vi "Main.vi"() -> ()   [LabVIEW 2020]
doc: "Use this template to build a simple state machine design pattern. Each state executes code and determines which state to transition to."
uses:
  controls/StateMachineVariables.ctl
  <vilib>/vision/Avi.llb/IMAQ AVI2 Refnum.ctl
  <vilib>/userDefined/High Color/IMAQdx.ctl
  <vilib>/vision/Deep Learning.llb/IMAQ DL Model Refnum.ctl
  <vilib>/vision/Image Controls.llb/IMAQ Image.ctl
  controls/State.ctl
panel:
  in  "Cluster":T1
  in  "Turn on the replay mode":bool=TRUE
  out "Replay mode":bool
  in  "?":T6(tab)
  in  "Camera Name":refnum<k21> caption="IMAQdx Session"
  out "fps cam":dbl
  out "height":u32
  out "width":u32
  in  "Start Frame Number":u32
  out "Actual frame":u32
  in  "Frame increment":i32=1
  in  "Video fps":u32=30
  in  "Video filename":string="test_moving2.avi"
  in  "Height":i32=1080
  in  "Width":i32=1920
  out "fps detection":dbl
  out "Distance":sgl(graph)
  # "SWITCH MODE BETWEEN\nCAMERA OR REPLAY"
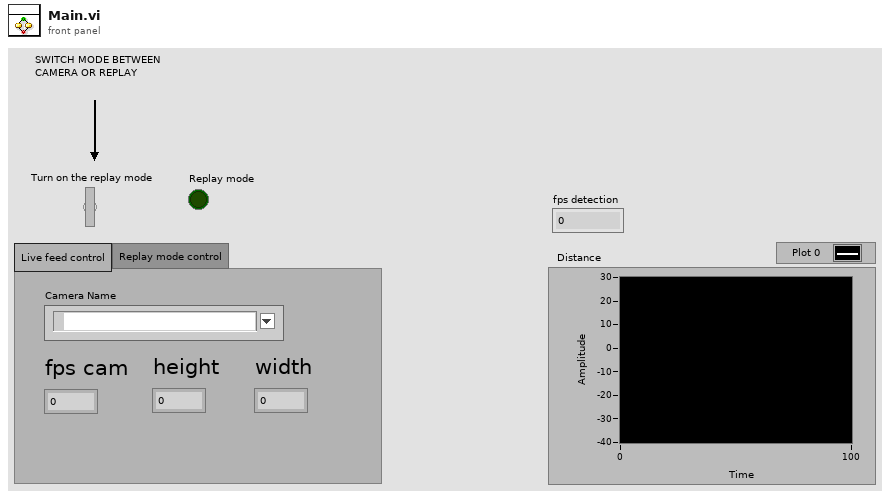
[diagram p1: front panel]
types:
  T1 = typedef "StateMachineVariables.ctl" = cluster{"AVI Refnum":T2, "Session ID":T3, "TensorFlow model refnum":T4, "Image refnum":T5, "VI path":path, "Horizontal distance":dbl, "Lateral distance":dbl, "Relative speed":dbl, "FPS":dbl}
  T2 = typedef "IMAQ AVI2 Refnum.ctl" = refnum<k20>
  T3 = typedef "IMAQdx.ctl" = refnum<k21>
  T4 = typedef "IMAQ DL Model Refnum.ctl" = refnum<k20>
  T5 = typedef "IMAQ Image.ctl" = refnum<image>
  T6 = enum32{"Live feed control", "Replay mode control"}
  T7 = typedef "State.ctl" = enum16{"Initialize VI path", "Initialize Video Session", "Initialize Cam session", "Initialize TensorFlow Model", "Initialize Image refnum", "Get video frame", "Get Cam frame", "Analyze image", "Update reaction space"}
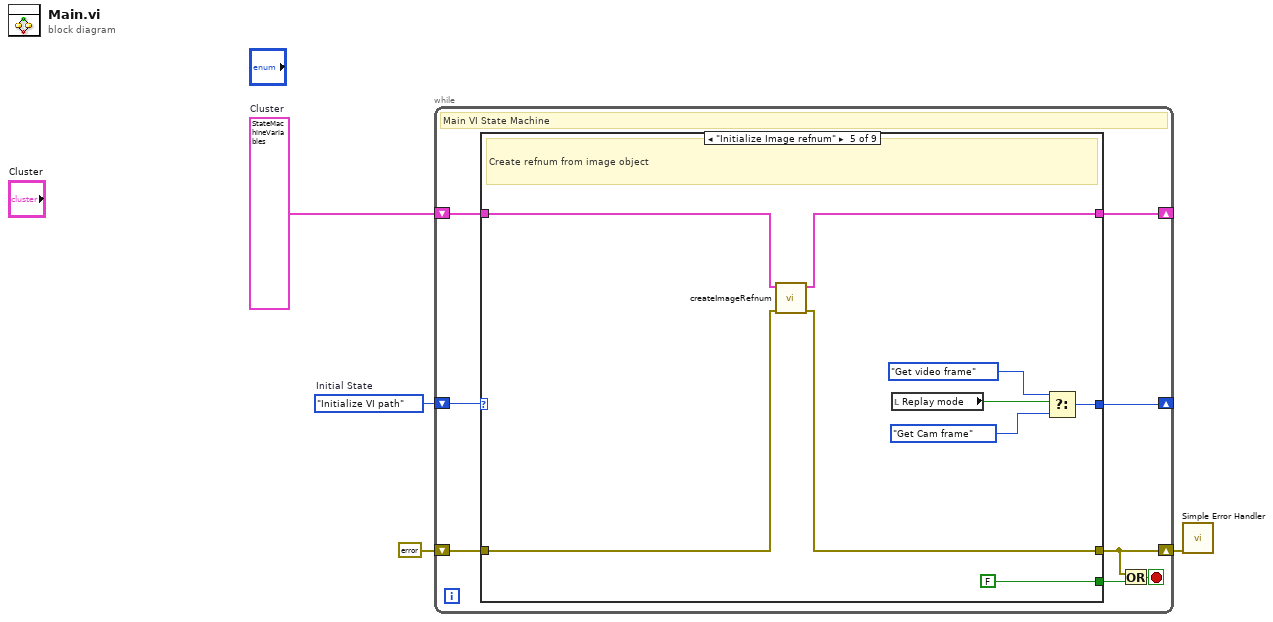
[diagram p0: block diagram]
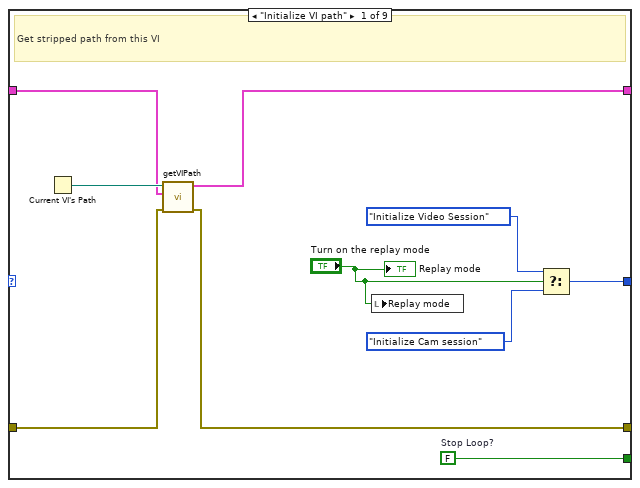
[diagram p2: hidden frame]
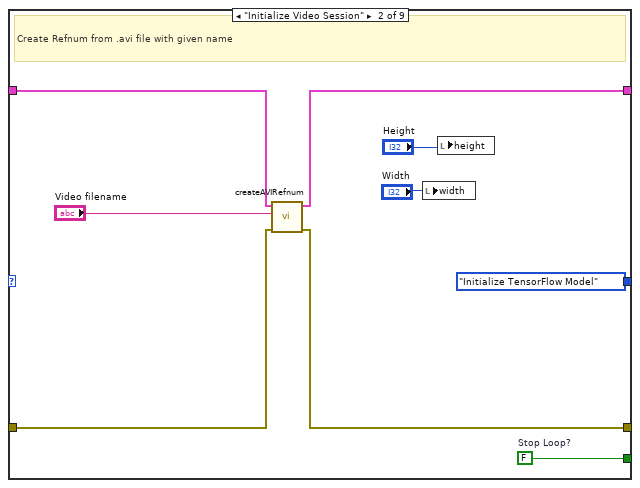
[diagram p3: hidden frame]
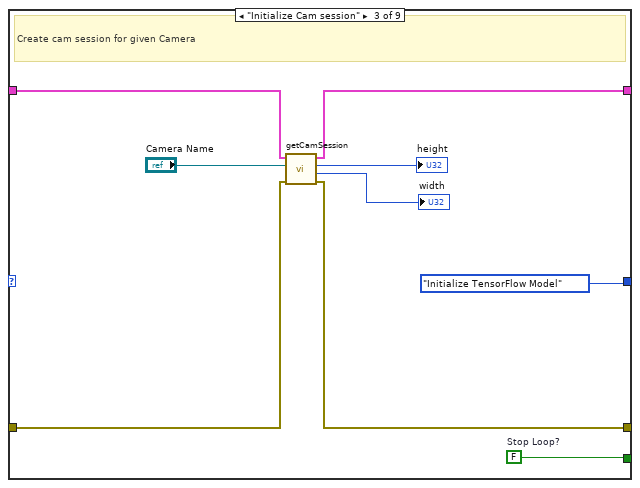
[diagram p4: hidden frame]
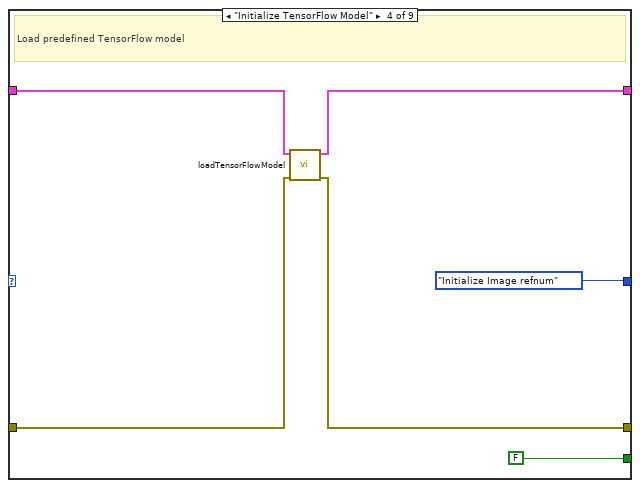
[diagram p5: hidden frame]
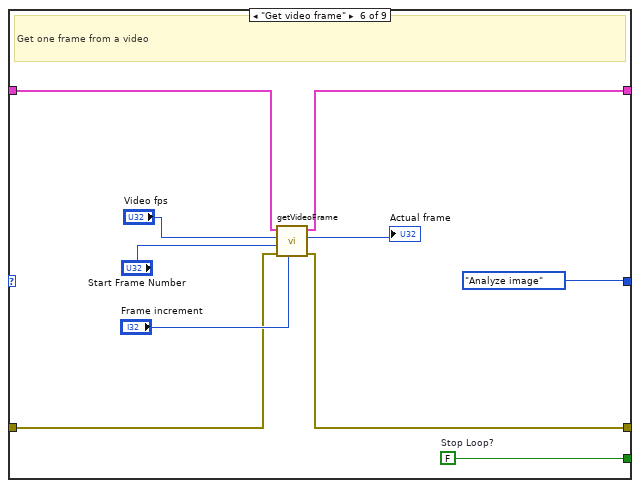
[diagram p6: hidden frame]
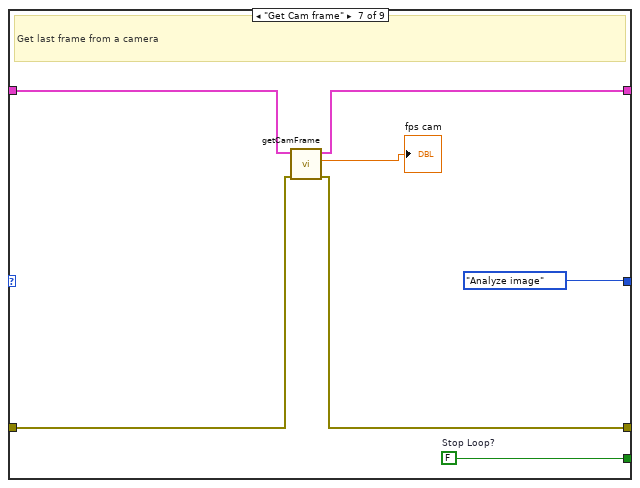
[diagram p7: hidden frame]
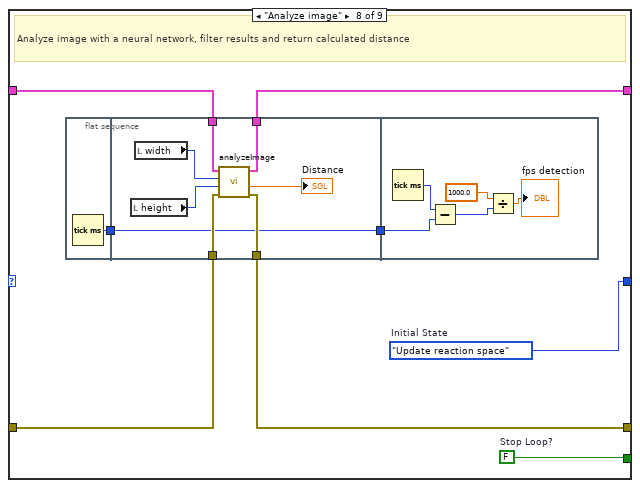
[diagram p8: hidden frame]
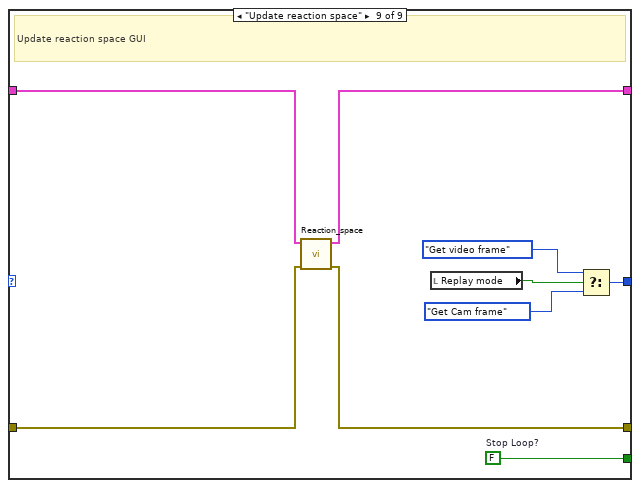
[diagram p9: hidden frame]
diagram:
  w2 = T1 {"AVI Refnum"=refnum, "Session ID"="", "TensorFlow model refnum"=refnum, "Image refnum"=refnum, "VI path"=path "", "Horizontal distance"=0.0, "Lateral distance"=0.0, "Relative speed"=0.0, "FPS"=0.0}  # Cluster
  w1 = State."Initialize VI path"  # Initial State
  n1 = while {
    shift-right: [w11] -> _
    shift-left: w2 -> [w12]
    shift-right: [w5] -> w3
    shift-left: errorcluster {"status"=FALSE, "code"=0, "source"=""} ("error constant") -> [w10]
    shift-right: [w7] -> _
    shift-left: w1 -> [w6]
    stop <- w8 stop-if-true
    # "Main VI State Machine"
    n2 = case shown="\"Initialize Image refnum\"" w6 {
      tunnel: [w15 State."Initialize TensorFlow Model" State."Initialize TensorFlow Model" State."Initialize Image refnum" w47 State."Analyze image" State."Analyze image" w75 w96] -> w7
      tunnel: [w22 w31 w34 FALSE ("Stop Loop?") FALSE ("Stop Loop?") w65 w67 w76 w99] -> w9
      tunnel: w12 -> [w20 w26 w39 w44 w54 w58 w72 w80 w103]
      tunnel: [w19 w25 w38 w43 w53 w59 w66 w79 w102] -> w11
      tunnel: w10 -> [w17 w24 w37 w41 w51 w60 w70 w78 w101]
      tunnel: [w18 w23 w36 w42 w52 w61 w69 w77 w100] -> w5
      frame "Initialize VI path" {
        w22 = FALSE  # Stop Loop?
        # "Get stripped path from this VI"
        n3 = Current VI's Path() -> (path=w21:path)
        n4 = call "getVIPath.vi"("error in"=w17, "Cluster in"=w20, "path"=w21) -> ("error out"=w18:errorcluster, "Cluster out"=w19:T1)  [unwired: 7 in]
        n5 = local write "Replay mode"("Turn on the replay mode") -> ()
        n6 = Select(t=State."Initialize Video Session", s="Turn on the replay mode", f=State."Initialize Cam session") -> (s? t:f=w15:T7)
        "Replay mode" <- "Turn on the replay mode"
      }
      frame "Initialize Video Session" {
        w31 = FALSE  # Stop Loop?
        # "Create Refnum from .avi file with given name"
        n7 = call "createAVIRefnum.vi"("error in"=w24, "Video filename"="Video filename", "Input cluster"=w26) -> ("error out"=w23:errorcluster, "Output cluster"=w25:T1)  [unwired: 7 in]
        n8 = local write "width"("Width") -> ()
        n9 = local write "height"("Height") -> ()
      }
      frame "Initialize Cam session" {
        w34 = FALSE  # Stop Loop?
        # "Create cam session for given Camera"
        n10 = call "getCamSession.vi"("error in"=w37, "Camera name"="Camera Name", "Input cluster"=w39) -> ("error out"=w36:errorcluster, "Width"=→"width":u32, "Height"=→"height":u32, "Output cluster"=w38:T1)  [unwired: 5 in]
      }
      frame "Initialize TensorFlow Model" {
        # "Load predefined TensorFlow model"
        n11 = call "loadTensorFlowModel.vi"("error in"=w41, "Input cluster"=w44) -> ("error out"=w42:errorcluster, "Output cluster"=w43:T1)  [unwired: 8 in]
      }
      frame "Initialize Image refnum" {
        # "Create refnum from image object"
        n12 = call "createImageRefnum.vi"("error in"=w51, "Output cluster in"=w54) -> ("error out"=w52:errorcluster, "Output cluster out"=w53:T1)  [unwired: 8 in]
        n13 = local read "Replay mode"() -> (w48:bool)
        n14 = Select(t=State."Get video frame", s=w48, f=State."Get Cam frame") -> (s? t:f=w47:T7)
      }
      frame "Get video frame" {
        w65 = FALSE  # Stop Loop?
        # "Get one frame from a video"
        n15 = call "getVideoFrame.vi"("Frame increment"="Frame increment", "error in (no error)"=w60, "Start Frame Number"="Start Frame Number", "Video fps"="Video fps", "Input cluster"=w58) -> ("error out"=w61:errorcluster, "Actual frame"=→"Actual frame":u32, "Output cluster"=w59:T1)  [unwired: 4 in]
      }
      frame "Get Cam frame" {
        w67 = FALSE  # Stop Loop?
        # "Get last frame from a camera"
        n16 = call "getCamFrame.vi"("error in (no error)"=w70, "Cluster"=w72) -> ("error out"=w69:errorcluster, "Acquired Frames per Second"=→"fps cam":dbl, "output cluster"=w66:T1)  [unwired: 7 in]
      }
      frame "Analyze image" {
        w76 = FALSE  # Stop Loop?
        w75 = State."Update reaction space"  # Initial State
        # "Analyze image with a neural network, filter results and return calculated distance"
        n17 = flat-sequence {
          tunnel: [w81] -> w74
          tunnel: w80 -> [w89]
          tunnel: [w88] -> w79
          tunnel: w78 -> [w84]
          tunnel: [w83] -> w77
          tunnel: w74 -> [w82]
          tunnel: [w82] -> w73
          tunnel: w73 -> [w91]
          frame #0 {
            n18 = Tick Count (ms)() -> (millisecond timer value=w81:u32)
          }
          frame #1 {
            n19 = local read "height"() -> (w85:u32)
            n20 = local read "width"() -> (w86:u32)
            n21 = call "analyzeImage.vi"("error in"=w84, "Height"=w85, "Width"=w86, "Input cluster"=w89) -> ("error out"=w83:errorcluster, "Output cluster"=w88:T1, "Distance"=→"Distance":sgl)  [unwired: 3 in, 2 out]
          }
          frame #2 {
            n22 = Tick Count (ms)() -> (millisecond timer value=w94:u32)
            n23 = Subtract(x=w94, y=w91) -> (x-y=w92:u32)
            n24 = Divide(x=1000.0, y=w92) -> (x/y=→"fps detection":dbl)
          }
        }
      }
      frame "Update reaction space" {
        w99 = FALSE  # Stop Loop?
        # "Update reaction space GUI"
        n25 = call "Reaction_space.vi"("error in"=w101, "Input cluster"=w103) -> ("error out"=w100:errorcluster, "Ouptut cluster"=w102:T1)  [unwired: 8 in]
        n26 = local read "Replay mode"() -> (w95:bool)
        n27 = Select(t=State."Get video frame", s=w95, f=State."Get Cam frame") -> (s? t:f=w96:T7)
      }
    }
    n28 = Or(x=w5, y=w9) -> (x .or. y?=w8:bool)
  }
  n29 = call <vilib>:"Simple Error Handler.vi"("error in (no error)"=w3) -> ()  [unwired: 4 in, 5 out]
